vi "像素操作.vi"() -> ()   [LabVIEW 2018]
uses:
  <vilib>/vision/NI_Vision_Development_Module.lvlib
panel:
  out "Image 2":T1(plugin-control)
  out "Image":T1(plugin-control)
  out "Pixels Line (I16)":i16[](array[numeric])
  out "error out":errorcluster
  out "Pixels (U8)":u8[](array[numeric])
  out "Pixel Value (U8)":u8
  in  "路径":path
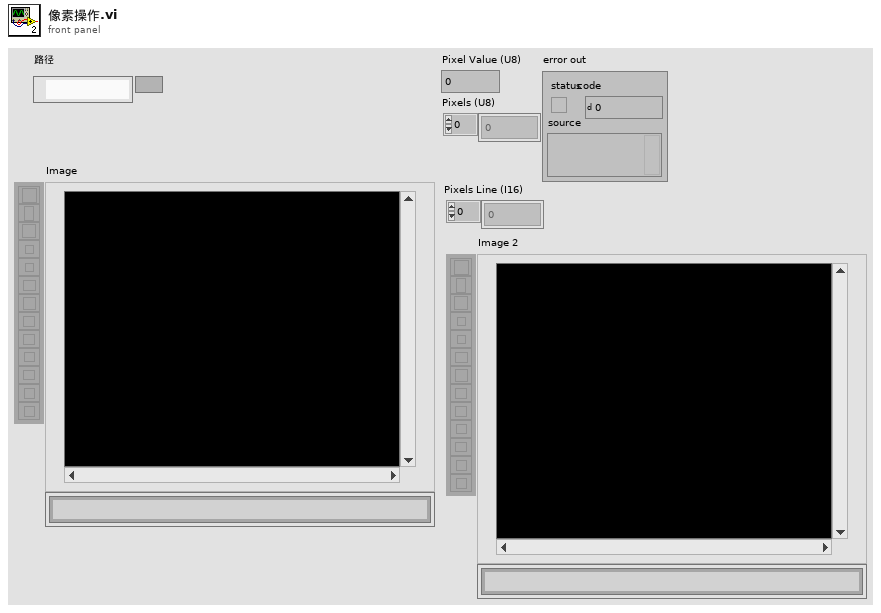
[diagram p1: front panel]
types:
  T1 = typedef "IMAQ Image.ctl" = refnum<image>
  T2 = typedef "Image Type" = u32
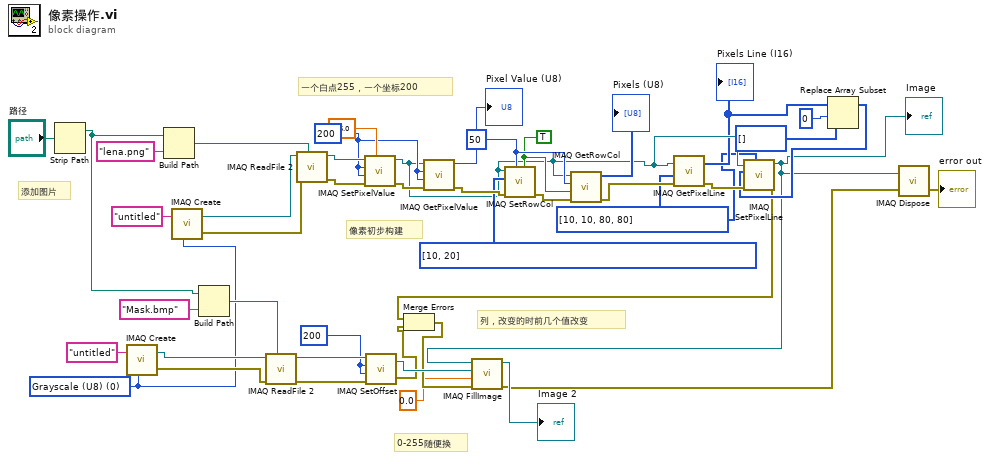
[diagram p0: block diagram]
diagram:
  w9 = 200 ("X Offset")
  w12 = T2 0 items=["Grayscale (U8)", "Grayscale (I16)", "Grayscale (SGL)", "Complex (CSG)", "RGB (U32)", "HSL (U32)", "RGB (U64)", "Grayscale (U16)"] ("Image Type")
  w19 = i32[] [10, 10, 80, 80] ("Line Coordinates")
  w30 = 50 ("Number")
  w29 = TRUE ("Row / Column (Row)")
  w35 = 200 ("X Coordinate")
  # "0-255随便换"
  # "添加图片"
  # "列，改变的时前几个值改变"
  # "像素初步构建"
  # "一个白点255，一个坐标200"
  n1 = Strip Path(path="路径") -> (stripped path=w17:path)  [unwired: 1 out]
  n2 = call "IMAQ Create"("Image Name"="untitled", "Image Type"=w12) -> ("New Image"=w15:T1, "error out"=w14:errorcluster)  [unwired: 3 in]
  n3 = Build Path(base path=w17, name or relative path="lena.png" ("名称或相对路径")) -> (appended path=w44:path)
  n4 = call "IMAQ Create"("Image Name"="untitled", "Image Type"=w12) -> ("New Image"=w41:T1, "error out"=w40:errorcluster)  [unwired: 3 in]
  n5 = Build Path(base path=w17, name or relative path="Mask.bmp" ("名称或相对路径")) -> (appended path=w16:path)
  n6 = call "IMAQ ReadFile 2"("File Path"=w16, "error in (no error)"=w14, "Image"=w15) -> ("error out"=w11:errorcluster, "Image Out"=w10:T1)  [unwired: 4 in, 3 out]
  n7 = call "IMAQ ReadFile 2"("File Path"=w44, "error in (no error)"=w40, "Image"=w41) -> ("error out"=w39:errorcluster, "Image Out"=w38:T1)  [unwired: 4 in, 3 out]
  n8 = call "IMAQ SetPixelValue"("Pixel Value"=sgl 255.0, "error in (no error)"=w39, "Y Coordinate"=w35, "X Coordinate"=w35, "Image"=w38) -> ("error out"=w36:errorcluster, "Image Out"=w25:T1)  [unwired: 5 in]
  n9 = call "IMAQ SetOffset"("error in (no error)"=w11, "Y Offset"=w9, "X Offset"=w9, "Image"=w10) -> ("error out"=w6:errorcluster, "Image Out"=w7:T1)
  n10 = call "IMAQ GetPixelValue"("Image"=w25, "X Coordinate"=w35, "Y Coordinate"=w35, "error in (no error)"=w36) -> ("Pixel Value (U8)"=→"Pixel Value (U8)":u8, "error out"=w33:errorcluster)  [unwired: 2 in, 3 out]
  n11 = call "IMAQ SetRowCol"("Row / Column (Row)"=w29, "Number"=w30, "error in (no error)"=w33, "Pixels (U8)"=u8[] [10, 20], "Image"=w25) -> ("error out"=w31:errorcluster)  [unwired: 5 in, 1 out]
  n12 = call "IMAQ GetRowCol"("Image"=w25, "Number"=w30, "Row / Column (Row)"=w29, "error in (no error)"=w31) -> ("Pixels (U8)"=→"Pixels (U8)":u8[], "error out"=w26:errorcluster)  [unwired: 2 in, 3 out]
  n13 = call "IMAQ GetPixelLine"("error in (no error)"=w26, "Line Coordinates"=w19, "Image"=w25) -> ("error out"=w24:errorcluster, "Pixels Line (I16)"=w23:i16[])  [unwired: 1 in, 3 out]
  "Pixels Line (I16)" <- w23
  n14 = Replace Array Subset(array=w23, new element=i16[] [] ("新元素/子数组"), index=0 ("索引")) -> (w20:i16[])
  n15 = call "IMAQ SetPixelLine"("Line Coordinates"=w19, "error in (no error)"=w24, "Pixels Line (U8)"=w20, "Image"=w25) -> ("error out"=w8:errorcluster, "Image Out"=w1:T1)  [unwired: 6 in]
  "Image" <- w1
  n16 = Merge Errors(w8, w6) -> (w5:errorcluster)
  n17 = call "IMAQ FillImage"("error in (no error)"=w5, "Pixel Value (U8, U16, I16, Float)"=sgl 0.0, "Image Mask"=w7, "Image"=w1) -> ("error out"=w2:errorcluster, "Image Out"=→"Image 2":T1)  [unwired: 6 in]
  n18 = call "IMAQ Dispose"("Image"=w1, "error in (no error)"=w2) -> ("error out"=→"error out":errorcluster)  [unwired: 4 in]
